vi "sendWaveform.vi"(2 "error in":errorcluster, 3 "connection ID":refnum<k5>, 4 "inputSignal":waveform(dbl)) -> (0 "error out":errorcluster, 1 "connection ID out":refnum<k5>)   [LabVIEW 2023]
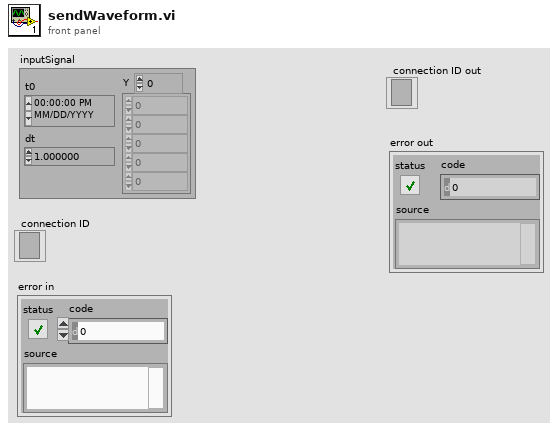
[diagram p1: front panel]
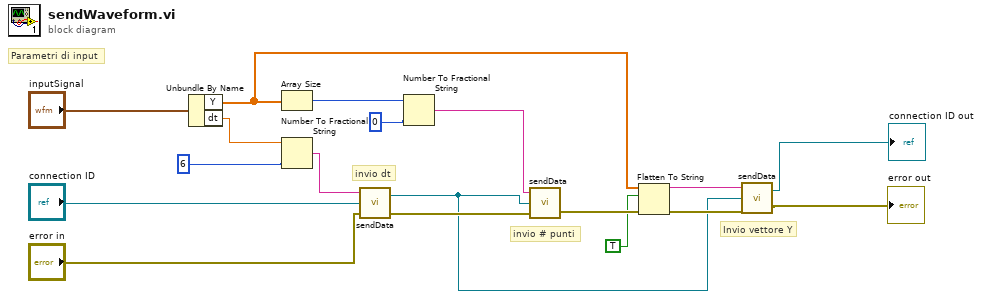
[diagram p0: block diagram]
diagram:
  # "Invio vettore Y"
  # "invio # punti"
  # "invio dt"
  # "Parametri di input"
  n1 = Unbundle By Name("inputSignal") -> ("Y"=w6:dbl[], "dt"=w17:dbl)
  n2 = Array Size(array=w6) -> (size(s)=w12:i32)
  n3 = Number To Fractional String(number=w17, precision (6)=i16 6) -> (F-format string=w15:string)  [unwired: 2 in]
  n4 = call "sendData.vi"("error in"="error in", "connection ID"="connection ID", "DATA"=w15) -> ("error out"=w9:errorcluster, "connection ID out"=w4:refnum<k5>)
  n5 = Number To Fractional String(number=w12, precision (6)=i16 0) -> (F-format string=w10:string)  [unwired: 2 in]
  n6 = call "sendData.vi"("error in"=w9, "connection ID"=w4, "DATA"=w10) -> ("error out"=w8:errorcluster)  [unwired: 1 out]
  n7 = Flatten To String(anything=w6, prepend array or string size? (T)=TRUE, error in (no error)=w8) -> (data string=w3:string, error out=w5:errorcluster)  [unwired: 1 in, 1 out]
  n8 = call "sendData.vi"("error in"=w5, "connection ID"=w4, "DATA"=w3) -> ("error out"=→"error out":errorcluster, "connection ID out"=→"connection ID out":refnum<k5>)
